vi "New Report Line.vi"(0 "report in":refnum<class "NI_report.lvclass">, 9 "number of lines (1)":i32=1, 11 "error in (no error)":errorcluster) -> (4 "report out":refnum<class "NI_report.lvclass">, 15 "error out":errorcluster)   [LabVIEW 2015, in "NI_report.lvclass"]
doc: "Starts a new line in the report."
uses:
  <vilib>/Utility/NIReport.llb/NI_report.lvclass
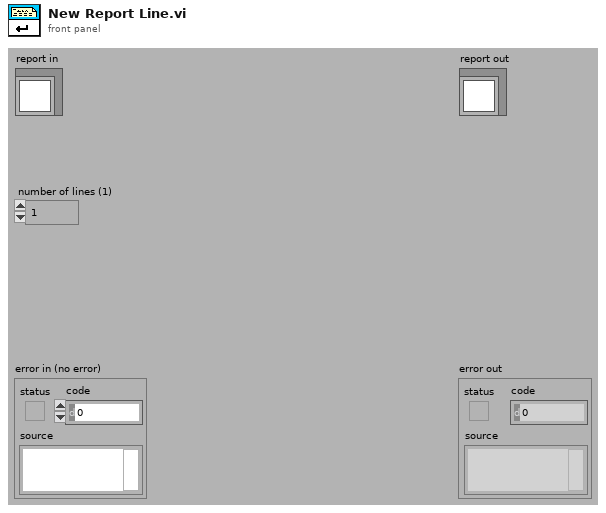
[diagram p1: front panel]
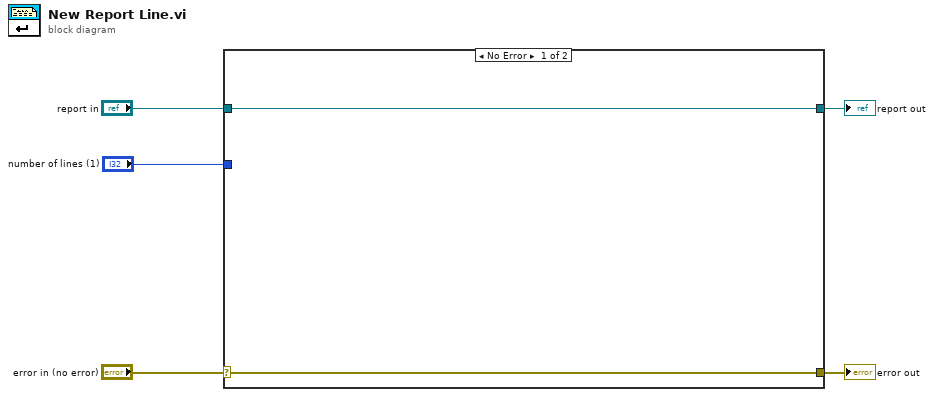
[diagram p0: block diagram]
diagram:
  n1 = case shown="No Error" "error in (no error)" {
    selector: "error in (no error)" -> [w6 w9]
    tunnel: [w6 w9] -> w4
    tunnel: [w7 w8] -> w2
    tunnel: "report in" -> [w7 w8]
    tunnel: "number of lines (1)" -> [_ _]
    frame No Error {
    }
    frame Error {
    }
  }
  "error out" <- w4
  "report out" <- w2
